vi "evaluate_gate.vi"(9 "acquiring?":bool, 10 "gate settings":T2, 11 "gate counters in":T1) -> (2 "pulse state out":bool, 3 "gate counters out":T1)   [LabVIEW 2010]
uses:
  common_typedefs/gate_parameters_cluster.ctl
  common_typedefs/gate_counters_cluster.ctl
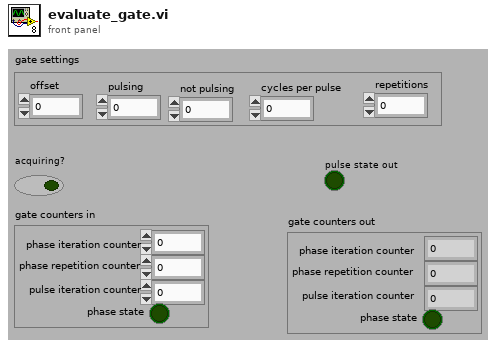
[diagram p1: front panel]
types:
  T1 = typedef "gate_counters_cluster.ctl" = cluster{"phase iteration counter":i64, "phase repetition counter":i64, "pulse iteration counter":i64, "phase state":bool}
  T2 = typedef "gate_parameters_cluster.ctl" = cluster{"offset":i64, "pulsing":i64, "not pulsing":i64, "cycles per pulse":i64, "repetitions":i64}
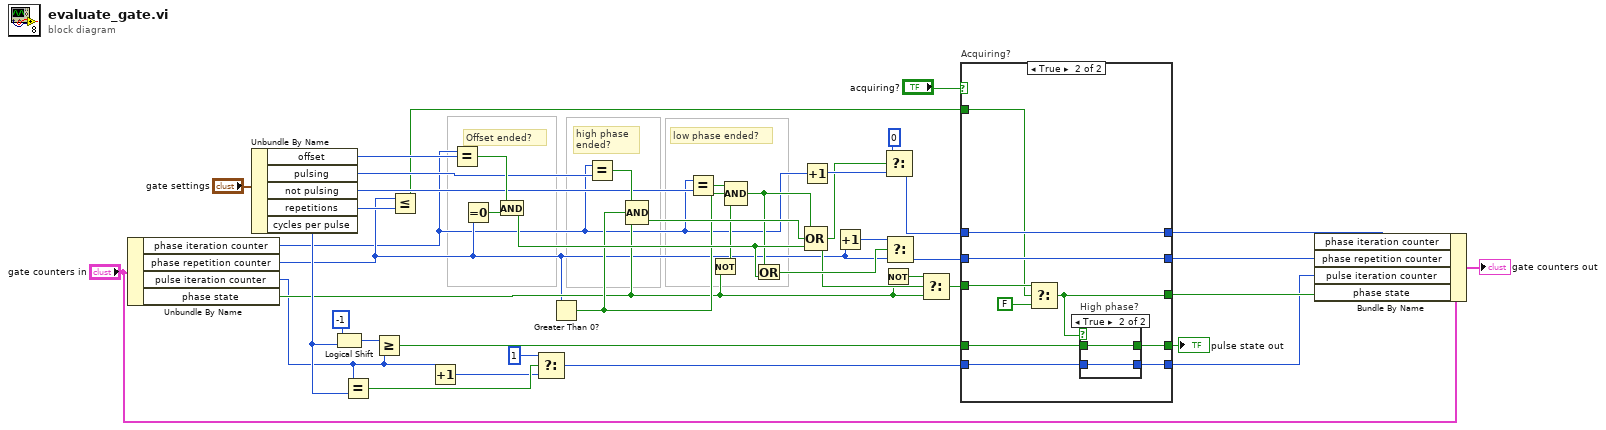
[diagram p0: block diagram]
diagram:
  # "low phase ended?"
  # "high phase ended?"
  # "Offset ended?"
  n1 = Unbundle By Name("gate counters in") -> ("phase iteration counter"=w7:i64, "phase repetition counter"=w9:i64, "pulse iteration counter"=w8:i64, "phase state"=w10:bool)
  n2 = Unbundle By Name("gate settings") -> ("offset"=w25:i64, "pulsing"=w37:i64, "not pulsing"=w30:i64, "repetitions"=w23:i64, "cycles per pulse"=w18:i64)
  n3 = Logical Shift(y=i8 -1, x=w18) -> (x << y=w19:i64)
  n4 = Equal?(x=w8, y=w18) -> (x = y?=w17:bool)
  n5 = Greater Or Equal?(x=w19, y=w8) -> (x >= y?=w13:bool)
  n6 = Less Or Equal?(x=w9, y=w23) -> (x <= y?=w22:bool)
  n7 = Increment(x=w8) -> (x+1=w16:i64)
  n8 = Equal?(x=w7, y=w25) -> (x = y?=w39:bool)
  n9 = Equal To 0?(x=w9) -> (x = 0?=w40:bool)
  n10 = And(x=w39, y=w40) -> (x .and. y?=w31:bool)
  n11 = Select(t=i64 1, s=w17, f=w16) -> (s? t:f=w14:i64)
  n12 = Greater Than 0?(x=w9) -> (x > 0?=w28:bool)
  n13 = Equal?(x=w7, y=w37) -> (x = y?=w41:bool)
  n14 = Compound Arithmetic op=AND(w41, w28, w10) -> (w32:bool)
  n15 = Equal?(x=w7, y=w30) -> (x = y?=w29:bool)
  n16 = Not(x=w10) -> (.not. x?=w11:bool)
  n17 = Compound Arithmetic op=AND(w29, w28, w11) -> (w24:bool)
  n18 = Or(x=w24, y=w31) -> (x .or. y?=w33:bool)
  n19 = Increment(x=w7) -> (x+1=w38:i64)
  n20 = Compound Arithmetic op=OR(w24, w32, w31) -> (w27:bool)
  n21 = Increment(x=w9) -> (x+1=w43:i64)
  n22 = Not(x=w10) -> (.not. x?=w26:bool)
  n23 = Select(t=i64 0, s=w27, f=w38) -> (s? t:f=w36:i64)
  n24 = Select(t=w43, s=w33, f=w9) -> (s? t:f=w35:i64)
  n25 = Select(t=w26, s=w27, f=w10) -> (s? t:f=w34:bool)
  n26 = case "Acquiring?" shown="True" "acquiring?" {
    tunnel: w36 -> [_ w53]
    tunnel: w35 -> [_ w54]
    tunnel: [_ w53] -> w3
    tunnel: [_ w54] -> w2
    tunnel: w34 -> [_ w51]
    tunnel: [_ w49] -> w5
    tunnel: w22 -> [_ w50]
    tunnel: [_ w45] -> w1
    tunnel: w14 -> [_ w47]
    tunnel: w13 -> [_ w48]
    tunnel: [_ w46] -> w12
    frame False {
    }
    frame True {
      n27 = Select(t=w51, s=w50, f=FALSE) -> (s? t:f=w49:bool)
      n28 = case "High phase?" shown="True" w49 {
        tunnel: w48 -> [_ w56]
        tunnel: w47 -> [_ w55]
        tunnel: [_ w56] -> w46
        tunnel: [_ w55] -> w45
        frame False {
        }
        frame True {
        }
      }
    }
  }
  "pulse state out" <- w12
  n29 = Bundle By Name(cluster="gate counters in", "phase iteration counter"=w3, "phase repetition counter"=w2, "pulse iteration counter"=w1, "phase state"=w5) -> (→"gate counters out":T1)
